vi "Manual XY input mode.vi"() -> (0 "error out":errorcluster, 1 "dataset names":string[](array[string]), 2 "file numbers":string[](array[string])=["1"], 3 "Data clusters":cluster{"array type (2D Dbl)":dbl[][]}[](array[cluster])=[{"array type (2D Dbl)"=[[0.0, 0.0], [0.0, 0.0], [0.0, 0.0], [18.81827, 0.30844], [18.35138, 0.31634], [17.87803, 0.3317], [17.40296, 0.34457], [16.91957, 0.35416], [16.54343, 0.36269], [16.06095, 0.37445], [15.57602, 0.39023], [15.0893, 0.40689], [14.6056, 0.42257], [14.11447, 0.43883], [13.63035, 0.45535], [13.13597, 0.47273], [12.64831, 0.49206], [12.17741, 0.51654], [11.68803, 0.53492], [11.215, 0.56209], [10.72076, 0.58603], [10.23037, 0.6157], [9.76891, 0.64471], [9.28946, 0.67794], [8.81078, 0.71328], [8.21509, 0.61292], [7.7324, 0.64903], [7.15451, 0.56693], [6.58079, 0.49252], [6.12455, 0.53112], [5.5621, 0.47305], [5.02753, 0.42776], [4.52093, 0.3925], [3.93975, 0.29851], [3.78387, 0.31388], [3.54704, 0.27516], [3.37637, 0.29195], [3.16443, 0.25393], [2.96481, 0.22427], [2.79286, 0.23987], [2.59221, 0.2134], [2.39643, 0.18865], [2.20831, 0.16658], [2.02395, 0.14868], [1.84703, 0.13218], [1.67515, 0.09644], [1.61029, 0.08046], [1.51098, 0.07147], [1.38897, 0.06622], [1.29939, 0.0627], [1.20588, 0.06488], [1.10809, 0.0647], [1.05747, 0.05618], [1.00991, 0.05378], [0.9693, 0.05571], [0.92684, 0.05043], [0.8743, 0.04901], [0.82101, 0.04098], [0.77652, 0.03748], [0.73085, 0.03536], [0.68851, 0.03129], [0.67289, 0.03234], [0.61459, 0.02901], [0.56683, 0.02536], [0.53192, 0.02179], [0.5115, 0.02178], [0.48294, 0.01822], [0.47519, 0.0181]]}], 4 "data names":string[](array[string]))   [LabVIEW 2021]
panel:
  in  "dataset name (option)":string="data"
  out "current data array":dbl[][](array[numeric])=[[0.0, 0.0], [0.0, 0.0], [0.0, 0.0], [18.81827, 0.30844], [18.35138, 0.31634], [17.87803, 0.3317], [17.40296, 0.34457], [16.91957, 0.35416], [16.54343, 0.36269], [16.06095, 0.37445], [15.57602, 0.39023], [15.0893, 0.40689], [14.6056, 0.42257], [14.11447, 0.43883], [13.63035, 0.45535], [13.13597, 0.47273], [12.64831, 0.49206], [12.17741, 0.51654], [11.68803, 0.53492], [11.215, 0.56209], [10.72076, 0.58603], [10.23037, 0.6157], [9.76891, 0.64471], [9.28946, 0.67794], [8.81078, 0.71328], [8.21509, 0.61292], [7.7324, 0.64903], [7.15451, 0.56693], [6.58079, 0.49252], [6.12455, 0.53112], [5.5621, 0.47305], [5.02753, 0.42776], [4.52093, 0.3925], [3.93975, 0.29851], [3.78387, 0.31388], [3.54704, 0.27516], [3.37637, 0.29195], [3.16443, 0.25393], [2.96481, 0.22427], [2.79286, 0.23987], [2.59221, 0.2134], [2.39643, 0.18865], [2.20831, 0.16658], [2.02395, 0.14868], [1.84703, 0.13218], [1.67515, 0.09644], [1.61029, 0.08046], [1.51098, 0.07147], [1.38897, 0.06622], [1.29939, 0.0627], [1.20588, 0.06488], [1.10809, 0.0647], [1.05747, 0.05618], [1.00991, 0.05378], [0.9693, 0.05571], [0.92684, 0.05043], [0.8743, 0.04901], [0.82101, 0.04098], [0.77652, 0.03748], [0.73085, 0.03536], [0.68851, 0.03129], [0.67289, 0.03234], [0.61459, 0.02901], [0.56683, 0.02536], [0.53192, 0.02179], [0.5115, 0.02178], [0.48294, 0.01822], [0.47519, 0.0181]]
  out "# of data set":i32=1
  in  "Done":bool=TRUE
  in  "add":bool
  out "XY Graph":T1(graph)={"array type (2D Dbl)"=[0.0, 0.0, 0.0, 18.81827, 18.35138, 17.87803, 17.40296, 16.91957, 16.54343, 16.06095, 15.57602, 15.0893, 14.6056, 14.11447, 13.63035, 13.13597, 12.64831, 12.17741, 11.68803, 11.215, 10.72076, 10.23037, 9.76891, 9.28946, 8.81078, 8.21509, 7.7324, 7.15451, 6.58079, 6.12455, 5.5621, 5.02753, 4.52093, 3.93975, 3.78387, 3.54704, 3.37637, 3.16443, 2.96481, 2.79286, 2.59221, 2.39643, 2.20831, 2.02395, 1.84703, 1.67515, 1.61029, 1.51098, 1.38897, 1.29939, 1.20588, 1.10809, 1.05747, 1.00991, 0.9693, 0.92684, 0.8743, 0.82101, 0.77652, 0.73085, 0.68851, 0.67289, 0.61459, 0.56683, 0.53192, 0.5115, 0.48294, 0.47519], "array type (2D Dbl)"=[0.0, 0.0, 0.0, 0.30844, 0.31634, 0.3317, 0.34457, 0.35416, 0.36269, 0.37445, 0.39023, 0.40689, 0.42257, 0.43883, 0.45535, 0.47273, 0.49206, 0.51654, 0.53492, 0.56209, 0.58603, 0.6157, 0.64471, 0.67794, 0.71328, 0.61292, 0.64903, 0.56693, 0.49252, 0.53112, 0.47305, 0.42776, 0.3925, 0.29851, 0.31388, 0.27516, 0.29195, 0.25393, 0.22427, 0.23987, 0.2134, 0.18865, 0.16658, 0.14868, 0.13218, 0.09644, 0.08046, 0.07147, 0.06622, 0.0627, 0.06488, 0.0647, 0.05618, 0.05378, 0.05571, 0.05043, 0.04901, 0.04098, 0.03748, 0.03536, 0.03129, 0.03234, 0.02901, 0.02536, 0.02179, 0.02178, 0.01822, 0.0181]}
  in  "Input window":string="18.81827\t0.30844\n18.35138\t0.31634\n17.87803\t0.3317\n17.40296\t0.34457\n16.91957\t0.35416\n16.54343\t0.36269\n16.06095\t0.37445\n15.57602\t0.39023\n15.0893\t0.40689\n14.6056\t0.42257\n14.11447\t0.43883\n13.63035\t0.45535\n13.13597\t0.47273\n12.64831\t0.49206\n9.28946\t0.67794\n8.81078\t0.71328\n8.21509\t0.61292\n7.7324\t0.64903\n7.15451\t0.56693\n6.58079\t0.49252"
  # "(1) Edit or Copy-Paste a single XY worksheet in the Input Window\n(2) Press  'Add'  to add the dataset\n(3) Repeat (1) and (2) until there is no more dataset\n(4) Press 'STOP'"
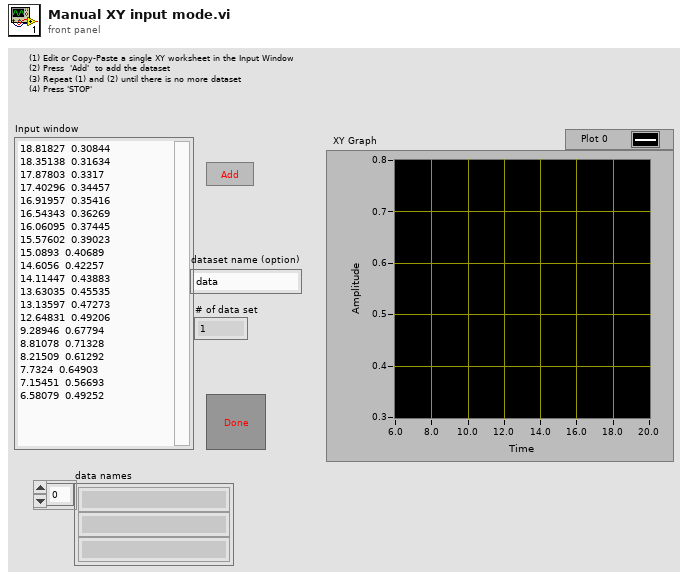
[diagram p1: front panel]
types:
  T1 = cluster{"array type (2D Dbl)":dbl[], "array type (2D Dbl)":dbl[]}
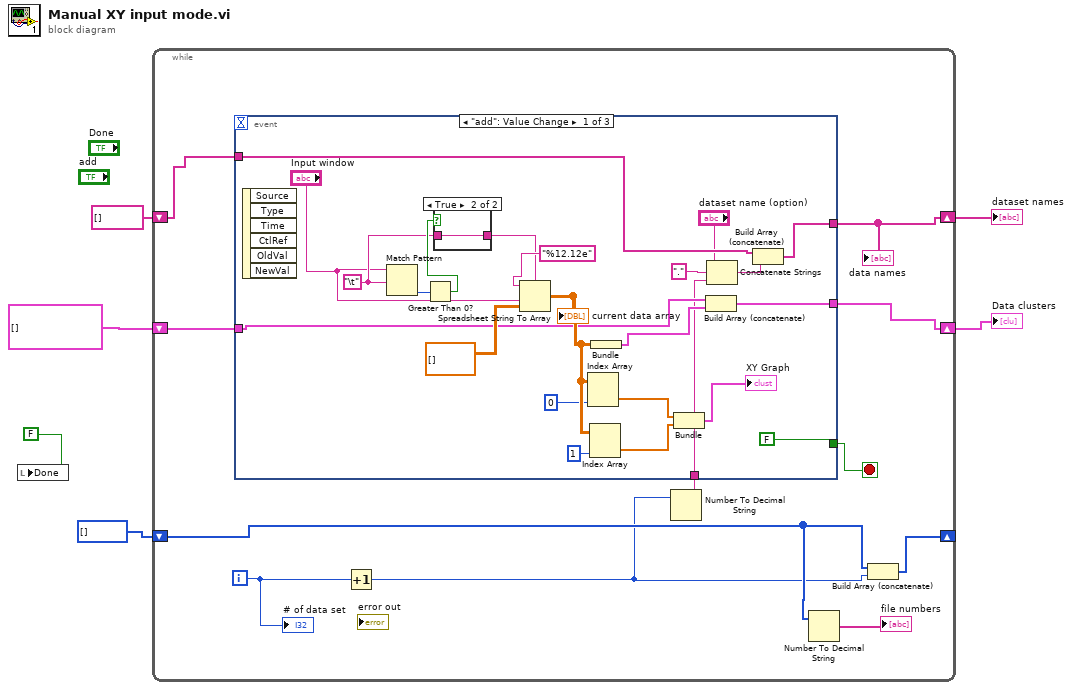
[diagram p0: block diagram]
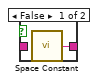
[diagram p2: hidden frame]
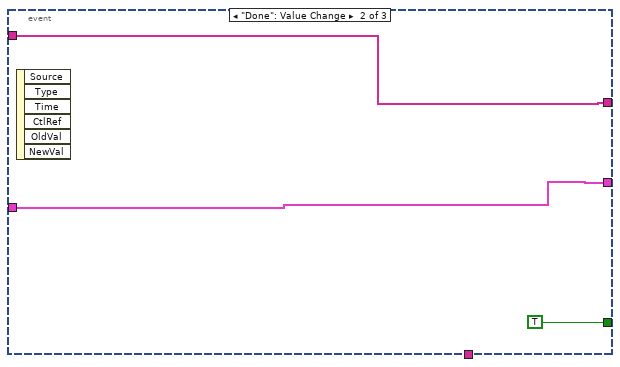
[diagram p3: hidden frame]
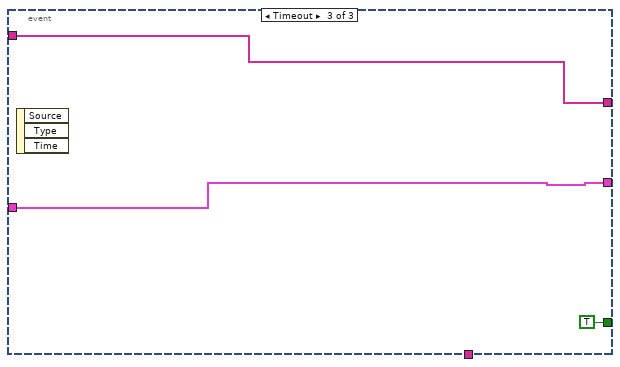
[diagram p4: hidden frame]
diagram:
  n1 = local write "Done"(FALSE ("End of Input")) -> ()
  n2 = while {
    shift-right: [w11] -> w3
    shift-left: cluster{"array type (2D Dbl)":dbl[][]}[] [] -> [w12]
    shift-right: [w17] -> _
    shift-left: i32[] [] -> [w14]
    shift-right: [w9] -> w1
    shift-left: string[] [] -> [w10]
    i -> [w16]
    stop <- w13 stop-if-true
    n3 = Increment(x=w16) -> (x+1=w8:i32)
    n4 = Number To Decimal String(number=w8) -> (decimal integer string=w7:string)  [unwired: 1 in]
    n5 = event shown="[0] \"add\": Value Change" {
      selector: _ -> [_ _ _]
      dyn-events: _ -> [_ _ _]
      timeout: _ -> [_ _ _]
      tunnel: [FALSE TRUE TRUE] -> w13
      tunnel: w12 -> [w26 w44 w48]
      tunnel: [w24 w44 w48] -> w11
      tunnel: [w23 w43 w47] -> w9
      tunnel: w10 -> [w22 w43 w47]
      tunnel: w7 -> [w19 _ _]
      event "add": Value Change {
        w29 = "\t"
        n6 = event-data() -> ()  [unwired: 1 in, 6 out]
        n7 = Match Pattern(string="Input window", regular expression=w29) -> (offset past match=w32:i32)  [unwired: 1 in, 3 out]
        n8 = Greater Than 0?(x=w32) -> (x > 0?=w31:bool)
        n9 = case shown="True" w31 {
          tunnel: [w41 w42] -> w30
          tunnel: w29 -> [_ w42]
          frame False {
            n10 = call <vilib>:"Space Constant.vi"() -> ("String"=w41:string)
          }
          frame True {
          }
        }
        n11 = Spreadsheet String To Array(delimiter (Tab)=w30, format string="%12.12e", spreadsheet string="Input window", array type (2D Dbl)=dbl[][] []) -> (array=w38:dbl[][])
        "current data array" <- w38
        n12 = Index Array(array=w38, index (col)=0 ("disabled index (col)")) -> (element=w35:dbl[])  [unwired: 1 in]
        n13 = Index Array(array=w38, index (col)=1 ("disabled index (col)")) -> (element=w34:dbl[])  [unwired: 1 in]
        n14 = Bundle("array type (2D Dbl)"=w38) -> (w25:cluster{"array type (2D Dbl)":dbl[][]})  [unwired: 1 in]
        n15 = Bundle("array type (2D Dbl)"=w35, "array type (2D Dbl)"=w34) -> (→"XY Graph":T1)  [unwired: 1 in]
        n16 = Build Array (concatenate)(w26, w25) -> (w24:cluster{"array type (2D Dbl)":dbl[][]}[])
        n17 = Concatenate Strings("dataset name (option)", "." ("string"), w19) -> (w20:string)
        n18 = Build Array (concatenate)(w22, w20) -> (w23:string[])
      }
      event "Done": Value Change {
        n19 = event-data() -> ()  [unwired: 1 in, 6 out]
      }
      event Timeout {
        n20 = event-data() -> ()  [unwired: 1 in, 3 out]
      }
    }
    "data names" <- w9
    n21 = Number To Decimal String(number=w14) -> (decimal integer string=→"file numbers":string[])  [unwired: 1 in]
    n22 = Build Array (concatenate)(w14, w8) -> (w17:i32[])
    "# of data set" <- w16
  }
  "Data clusters" <- w3
  "dataset names" <- w1
